vi "TEST ATAN2 and joystick functions.vi"() -> ()   [LabVIEW 2023]
uses:
  <vilib>/Rock Robotics/WPI/DriverStation/WPI_DriverStationAllianceInfo.ctl
  ctrl defs/ctrl FRONT FACE selector.ctl
  ctrl defs/ctrl DRIVING FRAME selector.ctl
panel:
  out "Array":T1(array[cluster])
  in  "current angle (deg)":dbl=5.0
  out "angle":dbl[](array[numeric])=[111.25110893724829, 150.25858148936936, 29.741418510630655, 68.7488910627517] format="%.4f"
  out "speed norm":dbl[](array[numeric])=[0.8999999999999999, 0.37570029466522775, 0.37570029466522775, 0.9] format="%.4f"
  in  "Vmax":dbl=0.9999999999999992 format="%#_13g"
  in  "MAX spin (rev/s)":dbl=0.7000000000000001 format="%#_13g"
  in  "drive frame":T2
  in  "HDG (deg)":dbl
  in  "front face":T3
  in  "Alliance":T4
  in  "sector width (deg)":dbl(ring)=60.0 items=["4-sectors"=90.0, "6-sectors"=60.0, "8-sectors"=45.0]
  in  "Sector":bool
  in  "Joystick":cluster{"Jx":dbl, "Jy":dbl, "Jr":dbl}[](array[cluster])=[{"Jx"=1.0, "Jy"=0.0, "Jr"=0.0}, {"Jx"=1.0, "Jy"=-1.0, "Jr"=0.0}, {"Jx"=0.0, "Jy"=-1.0, "Jr"=0.0}, {"Jx"=-1.0, "Jy"=-1.0, "Jr"=0.0}, {"Jx"=-1.0, "Jy"=0.0, "Jr"=0.0}, {"Jx"=-1.0, "Jy"=1.0, "Jr"=0.0}, {"Jx"=0.0, "Jy"=1.0, "Jr"=0.0}, {"Jx"=1.0, "Jy"=1.0, "Jr"=0.0}, {"Jx"=1.0, "Jy"=0.0, "Jr"=0.0}, {"Jx"=0.0, "Jy"=0.0, "Jr"=0.0}]
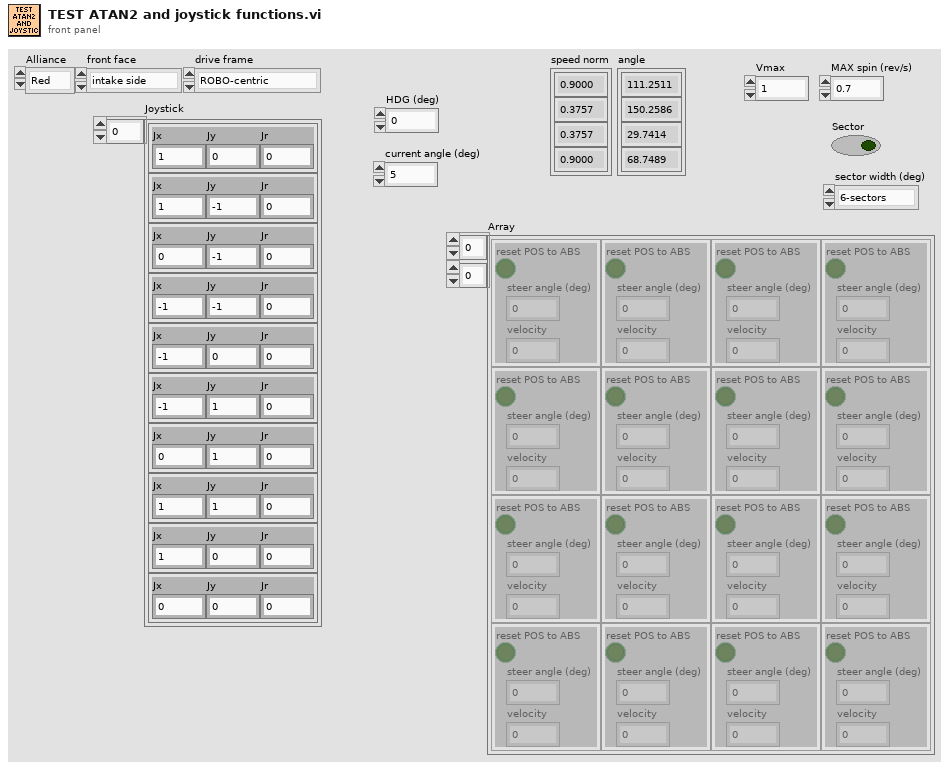
[diagram p1: front panel]
types:
  T1 = cluster{"reset POS to ABS":bool, "steer angle (deg)":dbl, "velocity":dbl}[][]
  T2 = typedef "ctrl DRIVING FRAME selector.ctl" = enum16{"ROBO-centric", "FLD-centric"}
  T3 = typedef "ctrl FRONT FACE selector.ctl" = enum16{"intake side", "shooter side"}
  T4 = typedef "WPI_DriverStationAllianceInfo.ctl" = enum16{"Red", "Blue", "Invalid"}
  T5 = cluster{"reset POS to ABS":bool, "steer angle (deg)":dbl, "velocity":dbl}
  T6 = typedef "ctrl driver input.ctl" = cluster{"Jx":dbl, "Jy":dbl, "Jr ":dbl, "R":dbl, "theta (deg)":dbl, "theta (rad)":dbl, "PARK":bool}
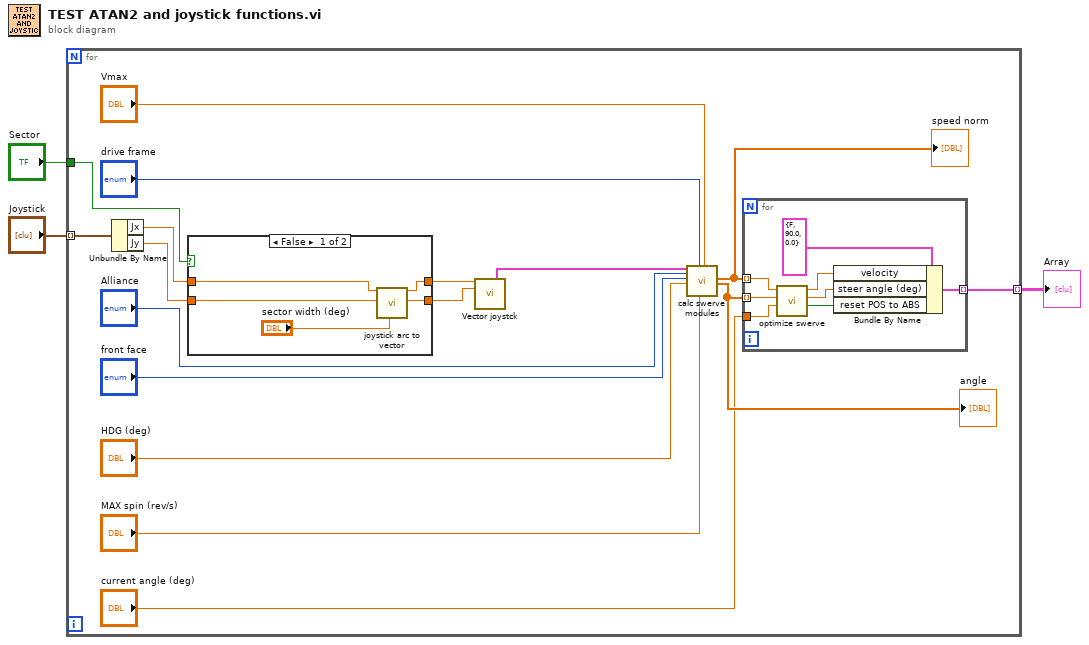
[diagram p0: block diagram]
diagram:
  n1 = for {
    tunnel: "Joystick" -> [w20] mode=indexing
    tunnel: "Sector" -> [w15]
    tunnel: [w5] -> w1 mode=indexing
    n2 = Unbundle By Name(w20) -> ("Jx"=w19:dbl, "Jy"=w18:dbl)
    n3 = case shown="False" w15 {
      tunnel: w19 -> [w33 w35]
      tunnel: w18 -> [w32 w34]
      tunnel: [w31 w35] -> w17
      tunnel: [w30 w34] -> w16
      frame False {
        n4 = call "joystick arc to vector.vi"("Jx"=w33, "Jy"=w32, "sector width (deg)"="sector width (deg)") -> ("Jx"=w31:dbl, "Jy"=w30:dbl)  [unwired: 13 in, 2 out]
      }
      frame True {
      }
    }
    n5 = call "Vector joystck.vi"("Jx input"=w17, "Jy input"=w16) -> ("output cluster"=w4:T6)  [unwired: 6 in, 7 out]
    n6 = call "calc swerve modules.vi"("DRIVER INPUT"=w4, "Alliance"="Alliance", "front face"="front face", "HDG (deg)"="HDG (deg)", "drive frame"="drive frame", "MAX spin (rev/s)"="MAX spin (rev/s)", "Vmax"="Vmax") -> ("speed norm"=w8:dbl[], "angle"=w7:dbl[])  [unwired: 10 in, 1 out]
    "speed norm" <- w8
    "angle" <- w7
    n7 = for {
      tunnel: w8 -> [w28] mode=indexing
      tunnel: w7 -> [w27] mode=indexing
      tunnel: "current angle (deg)" -> [w26]
      tunnel: [w21] -> w5 mode=indexing
      n8 = call "optimize swerve.vi"("current angle (deg)"=w26, "target angle (deg)"=w27, "velocity"=w28) -> ("reset POS to ABS"=w22:bool, "steer angle (deg)"=w23:dbl, "velocity"=w24:dbl)  [unwired: 5 in, 1 out]
      n9 = Bundle By Name(cluster=T5 {"reset POS to ABS"=FALSE, "steer angle (deg)"=90.0, "velocity"=0.0} ("Cluster"), "velocity"=w24, "steer angle (deg)"=w23, "reset POS to ABS"=w22) -> (w21:T5)
    }
  }
  "Array" <- w1
